vi "HSE Logger Custom Probe - DEBUG (String).vi"(11 "Callchain":string) -> (2 "Value String":string, 3 "Boolean":bool)   [LabVIEW 2016]
uses:
  HSE-Logger/hse-logger.lvlib
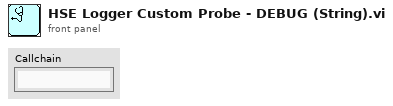
[diagram p1: front panel]
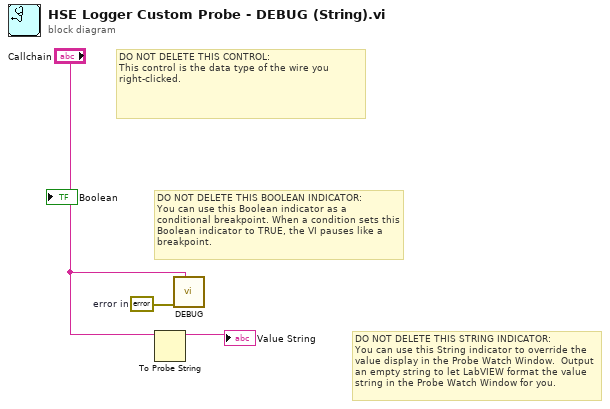
[diagram p0: block diagram]
diagram:
  w2 = errorcluster {"status"=FALSE, "code"=0, "source"=""}  # error in
  # "DO NOT DELETE THIS STRING INDICATOR: \nYou can use this String indicator to override the value display in the Probe Watch Window.  Output an empty string to let LabVIEW format the value string in the Probe Watch Window for you."
  # "DO NOT DELETE THIS BOOLEAN INDICATOR: \nYou can use this Boolean indicator as a conditional breakpoint. When a condition sets this Boolean indicator to TRUE, the VI pauses like a breakpoint."
  # "DO NOT DELETE THIS CONTROL: \nThis control is the data type of the wire you right-clicked."
  n1 = To Probe String(7:"Callchain") -> (3:→"Value String":string)  [unwired: 2 in, 1 out]
  n2 = call "DEBUG.vi"("Message"="Callchain", "error in"=w2) -> ()  [unwired: 9 in, 1 out]
